vi "method2.vi"(8 "error in (no error)":errorcluster, 10 "RefNum":i32, 11 "ProviderClass in":refnum<class "ProviderClass.lvclass">) -> (0 "error out":errorcluster, 2 "Boolean":bool, 3 "ProviderClass out":refnum<class "ProviderClass.lvclass">)   [LabVIEW 2019, in "lv-providershell-example3.lvlib" / "ProviderClass.lvclass"]
uses:
  ProviderClass.lvclass
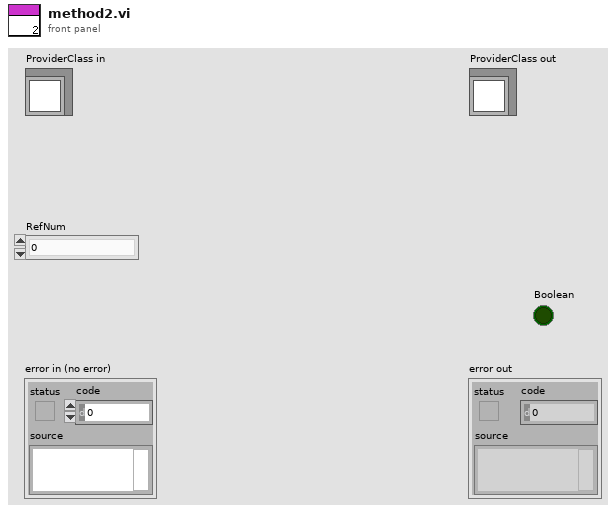
[diagram p1: front panel]
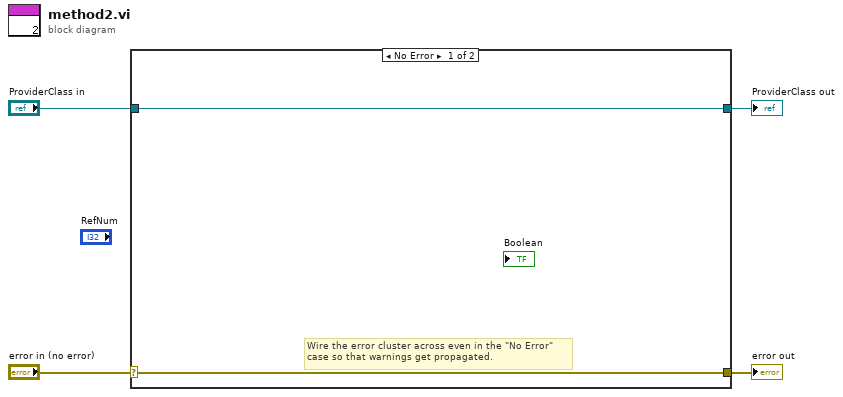
[diagram p0: block diagram]
diagram:
  n1 = case shown="No Error" "error in (no error)" {
    selector: "error in (no error)" -> [w5 w8]
    tunnel: [w5 w8] -> w3
    tunnel: [w6 w7] -> w1
    tunnel: "ProviderClass in" -> [w6 w7]
    frame No Error {
      # "Wire the error cluster across even in the \"No Error\"\ncase so that warnings get propagated."
    }
    frame Error {
    }
  }
  "error out" <- w3
  "ProviderClass out" <- w1
